vi "ODE_Template.vi"(0 "Reac Info":string[][](array[string])=[["Degradation_GFP", "", "false", "false", "Cell", "1", "GFP", "1.0", "true", "0", "", "", "0", "", "1", "kd", "0.0075"], ["Degradation_TetR", "", "false", "false", "Cell", "1", "TetR", "1.0", "true", "0", "", "", "0", "", "1", "kd", "0.0075"], ["Degradation_LacI", "", "false", "false", "Cell", "1", "LacI", "1.0", "true", "0", "", "", "0", "", "1", "kd", "0.0075"], ["R_abstracted_production_P1", "", "false", "false", "Cell", "0", "", "", "true", "1", "GFP", "10.0", "1", "LacI", "6", "RNAP, ng__P1, Ko__P1, ko__P1, nc__LacI_P1, Kr__LacI_P1", "30.0, 2.0, 0.033, 0.05, 2.0, 0.5"], ["R_abstracted_production_P2", "", "false", "false", "Cell", "0", "", "", "true", "1", "GFP", "10.0", "1", "TetR", "6", "RNAP, ng__P2, Ko__P2, ko__P2, nc__TetR_P2, Kr__TetR_P2", "30.0, 2.0, 0.033, 0.05, 2.0, 0.5"]], 1 "Ex_Mod_IDs":string[](array[string])=["LacI", "TetR"], 2 "Idx of Mod in Sp IDs":i32[](array[numeric])=[1, 4], 5 "Math Expressions":string[](array[string])=["kd*GFP", "kd*TetR", "kd*LacI", "ko__P1*ng__P1*Ko__P1*RNAP/(1+Ko__P1*RNAP+(Kr__LacI_P1*LacI)^nc__LacI_P1)", "ko__P2*ng__P2*Ko__P2*RNAP/(1+Ko__P2*RNAP+(Kr__TetR_P2*TetR)^nc__TetR_P2)"], 7 "Species Info":string[][](array[string])=[["GFP", "", "Cell", "0.0", "NaN", "", "true", "false", "false", "null"], ["LacI", "", "Cell", "0.0", "NaN", "", "true", "true", "false", "null"], ["P1", "", "Cell", "2.0", "NaN", "", "true", "false", "false", "null"], ["P2", "", "Cell", "2.0", "NaN", "", "true", "false", "false", "null"], ["TetR", "", "Cell", "0.0", "NaN", "", "true", "true", "false", "null"]], 9 "Parameter info":string[][](array[string])=[["ko_r", "Reverse RNAP binding rate", "1.0", "", "true"], ["nr", "Initial RNAP count", "30.0", "", "true"], ["np", "Stoichiometry of production", "10.0", "", "true"], ["kr_r", "Reverse repression binding rate", "1.0", "", "true"], ["ka_f", "Forward activation binding rate", "0.0033", "", "true"], ["kecdiff", "Extracellular diffusion rate", "1.0", "", "true"], ["ko", "Open complex production rate", "0.05", "", "true"], ["kmdiff_f", "Forward membrane diffusion rate", "1.0", "", "true"], ["kecd", "Extracellular degradation rate", "0.005", "", "true"], ["kc_r", "Reverse complex formation rate", "1.0", "", "true"], ["kr_f", "Forward repression binding rate", "0.5", "", "true"], ["ka_r", "Reverse activation binding rate", "1.0", "", "true"], ["nc", "Stoichiometry of binding", "2.0", "", "true"], ["kao_r", "Reverse activated RNAP binding rate", "1.0", "", "true"], ["kd", "Degradation rate", "0.0075", "", "true"], ["kb", "Basal production rate", "1.0E-4", "", "true"], ["ng", "Initial promoter count", "2.0", "", "true"], ["ka", "Activated production rate", "0.25", "", "true"], ["kao_f", "Forward activated RNAP binding rate", "1.0", "", "true"], ["kmdiff_r", "Reverse membrane diffusion rate", "0.01", "", "true"], ["ko_f", "Forward RNAP binding rate", "0.033", "", "true"], ["kc_f", "Forward complex formation rate", "0.05", "", "true"], ["High", "", "120.0", "", "true"], ["HighTime", "", "1000.0", "", "true"], ["HighTime2", "", "2000.0", "", "true"]], 11 "Local Parameter Info":string[][](array[string])=[["kd", "0.0075"], ["kd", "0.0075"], ["kd", "0.0075"], ["RNAP", "30.0"], ["ng__P1", "2.0"], ["Ko__P1", "0.033"], ["ko__P1", "0.05"], ["nc__LacI_P1", "2.0"], ["Kr__LacI_P1", "0.5"], ["RNAP", "30.0"], ["ng__P2", "2.0"], ["Ko__P2", "0.033"], ["ko__P2", "0.05"], ["nc__TetR_P2", "2.0"], ["Kr__TetR_P2", "0.5"]]) -> ()   [LabVIEW 2014]
uses:
  Modifier Control.ctl
  ODE Simulation Parameters.ctl
  <vilib>/Simulation/Implementation/Shared/SIM Continuous Solvers.ctl
  Event Info.ctl
  <vilib>/Utility/error.llb/DialogType.ctl
  Stop ODE.vi
  Sim status.vi
  Trigger Status Bar.vi
  <vilib>/Utility/file.llb/Write To Spreadsheet File (string).vi
  <vilib>/regexp/Match Regular Expression.xnode
panel:
  out "ScrSht Path":path
  out "loop":i32
  out "Rest_Sp_IDs":string[](array[string])
  out "Sp_Init_Amnt":string[](array[string])
  out "Fn Arg Cnt":string[](array[string])
  out "Functions":string[][](array[string])
  out "FuncCnt":i32
  out "Status update":string
  out "Trig Status":bool
  out "Comp IDs":string[](array[string])
  out "hasOnlySubstanceUnits":string[](array[string])
  out "Math-w/-ch-VarID":string[](array[string])
  out "LP_IDs":string[](array[string])
  out "Pr_Id_Arr":string[](array[string])
  out "Sp IDs":string[](array[string])
  out "Cap Cnt":i32
  out "Plot Legends":string[](array[string])
  out "ModTimeSym":string
  out "CompSize":string[](array[string])
  out "CompID":string[](array[string])
  out "Comp Def":string[][](array[string])
  out "Rules":string[][](array[string])
  out "RulesCnt":i32
  in  "Run":bool
  in  "Reset":bool
  in  "Stop Main":bool
  out "Sp_Name":string[](array[string])
  out "Nxt Sp State (N)":dbl[](array[numeric])
  out "T":dbl[](array[numeric])
  out "AppPath":string
  out "path":path
  in  "Shut Down":bool
  out "Sim Data":cluster{"times":dbl[], "outputs":dbl[][]}
  out "Rest_Sp_Init_Amnt":string[](array[string])
  in  "Simulation Parameters":T1={"Initial Time"=0.0, "Final Time"=20.0, "Time Step"=0.1, "Absolute Tolerance"=0.001, "Relative Tolerance"=1e-06, "Type of Continuous Solver"=enum."Runge-Kutta 45 (variable)", "Discrete Time Step"=2.0, "Minimum Time Step"=1e-06, "Maximum Time Step"=1.0, "Initial Time Step"=0.1} {"Initial Time Step" min=0.0; "Maximum Time Step" min=0.0; "Minimum Time Step" min=0.0; "Discrete Time Step" min=0.0; "Relative Tolerance" min=0.0; "Absolute Tolerance" min=0.0; "Time Step" min=0.0}
  in  "SP_for_ODE_Init_Amnt":string[](array[string])
  out "Out_X_for_ODE":string[](array[string])
  out "Out_Tot_Param":string[](array[string])
  out "Out_ODE":string[](array[string])
  in  "Model Name":string="nand_RB"
  out "Sp Ids":string[](array[string])
  out "XY Graph":cluster{"T":dbl[], dbl[]}[](graph)
  out "Nxt Sp State (S)":string[](array[string])
  out "Init Sp State (S)":string[](array[string])
  out "All Param Names":string[](array[string])
  out "Equations":string[](array[string])
  out "Init Sp State (N)":dbl[](array[numeric])
  out "All Param Vals":string[](array[string])
  out "All Param IDs":string[](array[string])
  out "New Total Pr IDs":string[](array[string])
  in  "Event Info":T3
  out "All Variables":string[](array[string])
  out "Math Assign":string[](array[string])
  out "Triggering Math":string[](array[string])
  in  "External Modifiers":T4[](array[typedef]) {"Dial" scale=0.0..100.0 scale format="%#_3g"}
  in  "Del events after \nexecution":bool
  in  "Capture Graph":bool caption="Save Data 2"
  in  "Save Data":bool
  in  "Sim Param":bool
  out "All Param Values":string[](array[string])
  out "Status":string
  in  "Events Info":string[][](table)=[["event0", "true", "true", "true", "t >= HighTime", "TetR = High"], ["event1", "true", "true", "true", "t >= HighTime2", "LacI = High"]]
  out "DataLog":path
  out "decimal integer string":string
  out "Horizontal Progress Bar":u8(slide) scale=0.0..100.0
  # "Virtual Laboratory Instrument for ODE Simulations"
  # "Powered By"
  # "Model Parameters"
  # "Global Parameters"
  # "Local Parameters"
  # "ID"
  # "Name"
  # "Value"
  # "ID"
  # "Value"
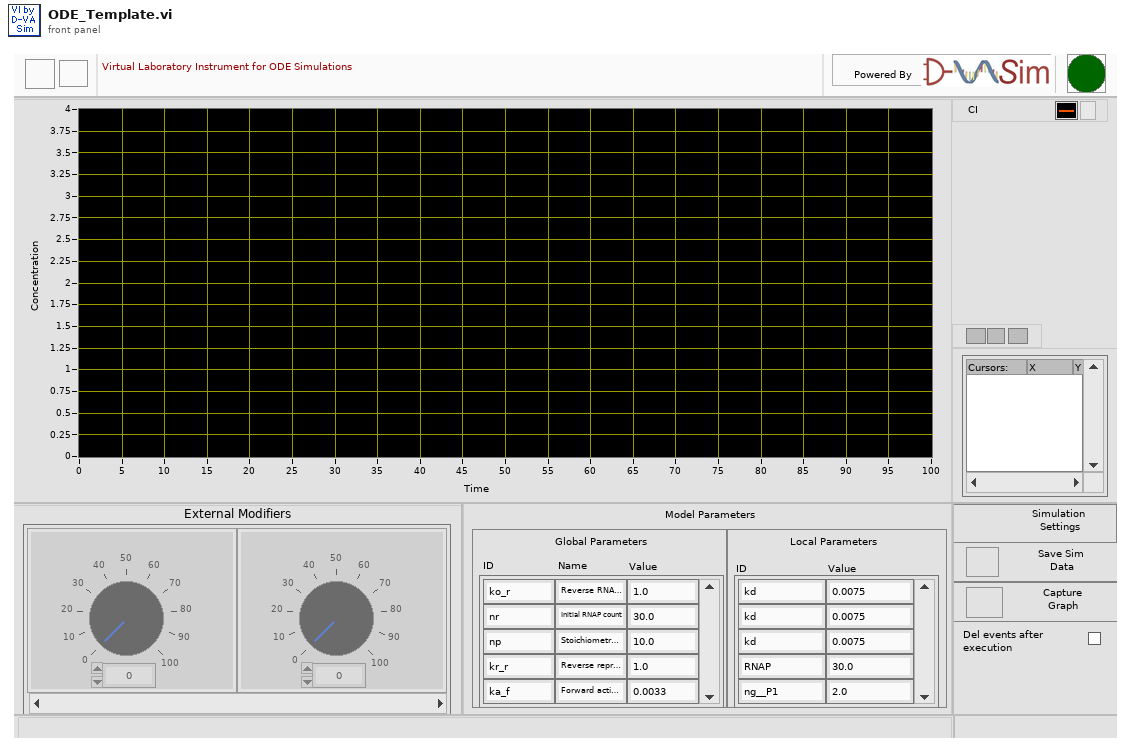
[diagram p1: front panel]
types:
  T1 = typedef "ODE Simulation Parameters.ctl" = cluster{"Initial Time":dbl, "Final Time":dbl, "Time Step":dbl, "Absolute Tolerance":dbl, "Relative Tolerance":dbl, "Type of Continuous Solver":T2, "Discrete Time Step":dbl, "Minimum Time Step":dbl, "Maximum Time Step":dbl, "Initial Time Step":dbl}
  T2 = typedef "SIM Continuous Solvers.ctl" = enum16{"Runge-Kutta 1 (Euler)", "Runge-Kutta 2", "Runge-Kutta 3", "Runge-Kutta 4", "Runge-Kutta 23 (variable)", "Runge-Kutta 45 (variable)", "BDF (variable)", "Adams-Moulton (variable)", "Rosenbrock (variable)", "Discrete States Only"}
  T3 = typedef "Event Info.ctl" = cluster{"Math Var":string[], "Math Op":string[], "Math Val":string[], "Assign Var":string[][], "Assign Op":string[][], "Assign Val":string[][], "Var Idx":i32[], "Assign Var Idx":i32[][], "Delay":string[], "Priority":string[]}
  T4 = typedef "Modifier Control.ctl" = cluster{"Dial":dbl, "String 2":string}
  T5 = enum8{"Enabled", "Disabled", "Disabled and Grayed Out"}
  T6 = typedef "DialogType.ctl" = u16
  T7 = typedef "Model Information.ctl" = cluster{"ID":string, "Name":string, "Substance Units":string, "Time Units":string, "Volume Units":string, "Area Units":string, "Length Units":string, "Extent Units":string, "Conversion Factor":string, "Model Components":string}
  T8 = cluster{"Model Info":T7, "SpCnt":i32, "Species Info":string[][], "Pr_Cnt":i32, "Parameter info":string[][], "ReacCnt":i32, "Reaction Info":string[][], "Math Expressions":string[][], "EventsCnt":i32, "Event Info":string[][], "UnitsDefCnt":i32, "Units Def":string[][], "CompCnt":i32, "Comp Def":string[][], "Mod_ID":string[], "Mod_Idx":i32[], "RulesCnt":i32, "Rules":string[][], "FuncCnt":i32, "Functions":string[][], "InitAssign Cnt":i32, "Init Assigns":string[][], "ConstraintsCnt":i32, "Constraints":string[][], "Fn Arg Cnt":string[]}
  T9 = cluster{"Reac Info":string[], "Reac Info":string[], "Reac Info":string[], "Math Expressions":string[], "Reac Info":string[], "Species Info":string[], "Sp IDs":string[], "Math-w/-ch-VarID":string[], "hasOnlySubstanceUnits":string[], "Comp IDs":string[]}
  T10 = cluster{"SP-for-ODE":string[], "Reac Info":string[], "Sp IDs":string[], "Species Info":string[], string[], "Reac Info":string[], "Reac Info":string[]}
  T11 = cluster{"Ex_Mod_IDs":string[], "Ex_Mod_IDs+Names":string[], "Ex_Mod_Init_Amnt":string[], "Rest_Sp_IDs ":string[], "Rest_Sp_IDs+Names":string[], "Rest_Sp_Init_Amnt":string[], "SP_for_ODE_Init_Amnt":string[], "Sp_for_ODE+Names":string[]}
  T12 = enum32{"invalid app kind", "Development System", "Run Time System", "Student Edition", "Embedded LabVIEW", "Evaluation", "Custom"}
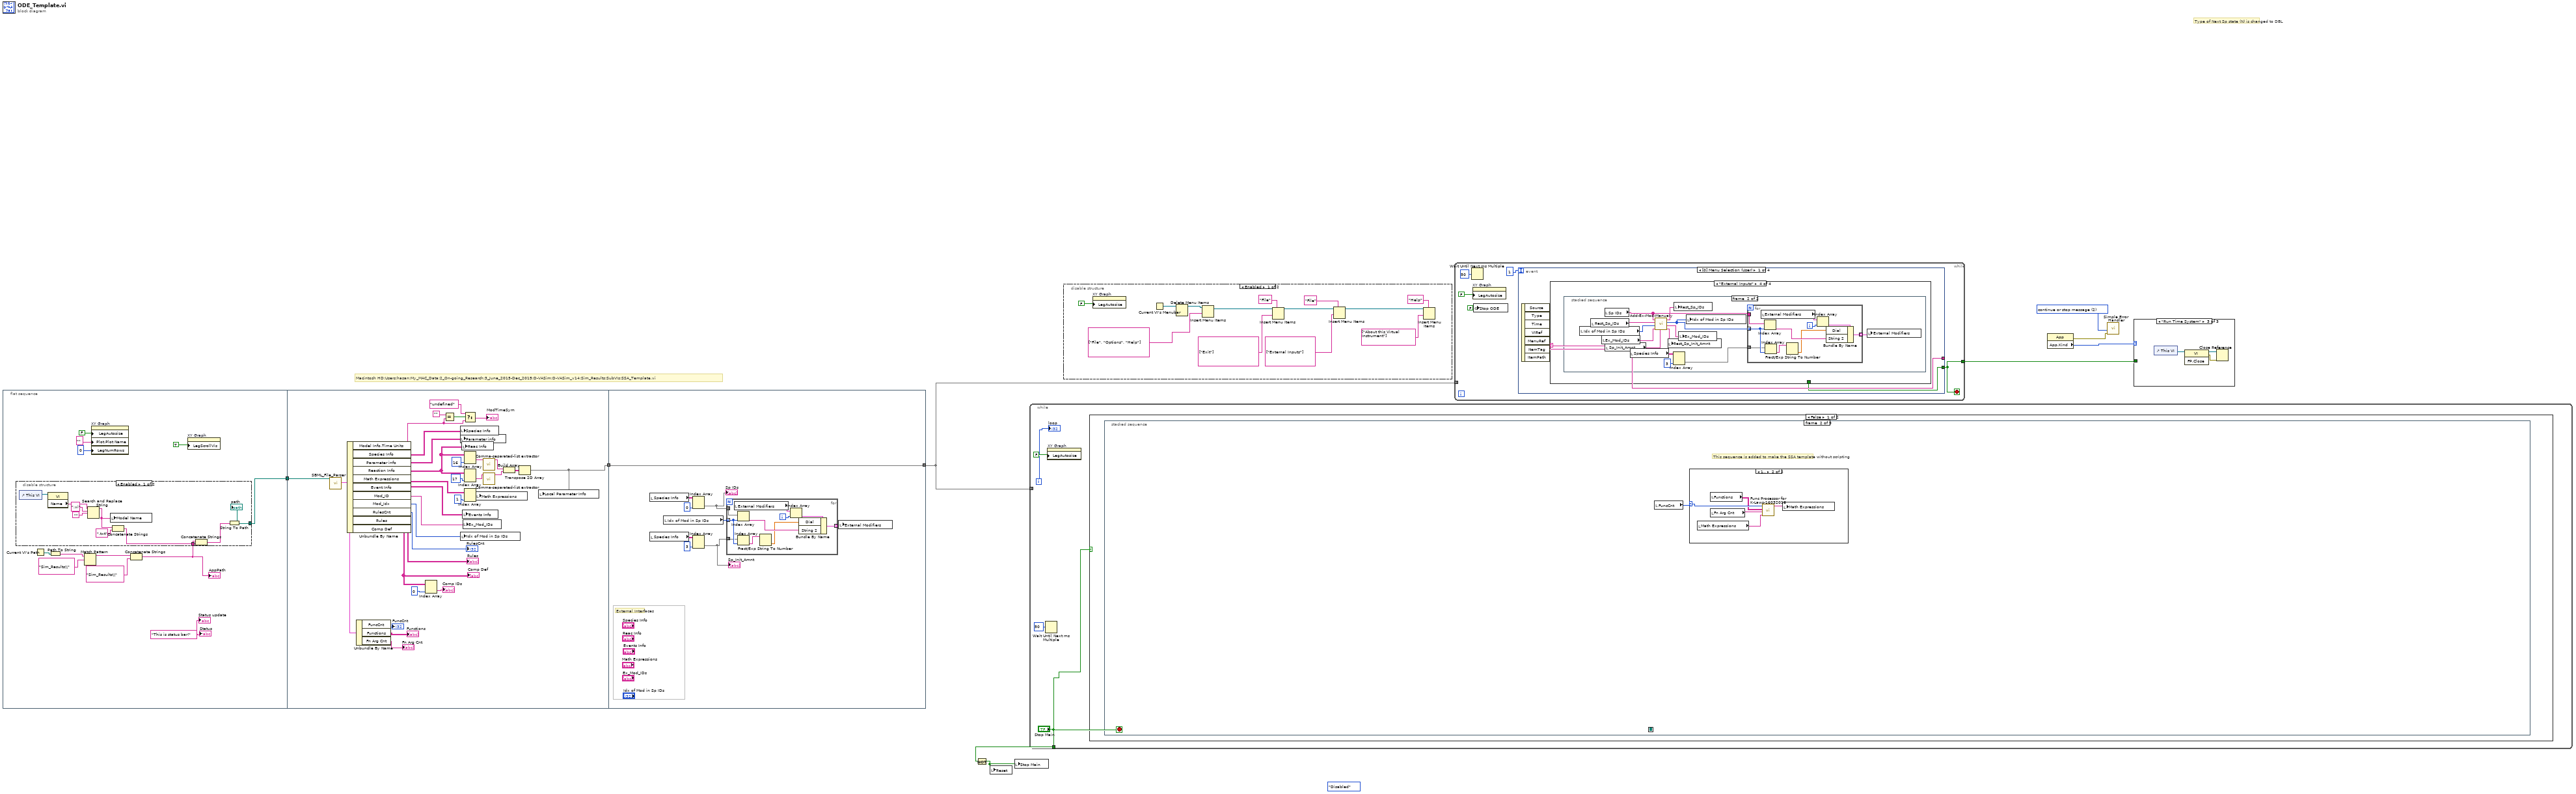
[diagram p0: block diagram]
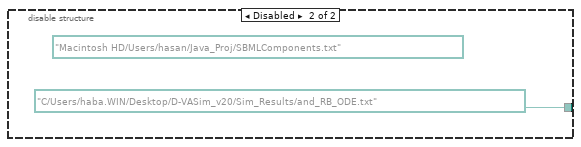
[diagram p2: hidden frame]
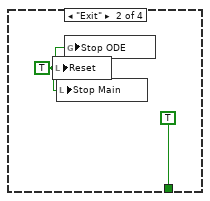
[diagram p7: hidden frame]
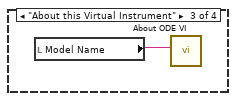
[diagram p8: hidden frame]
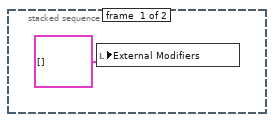
[diagram p9: hidden frame]
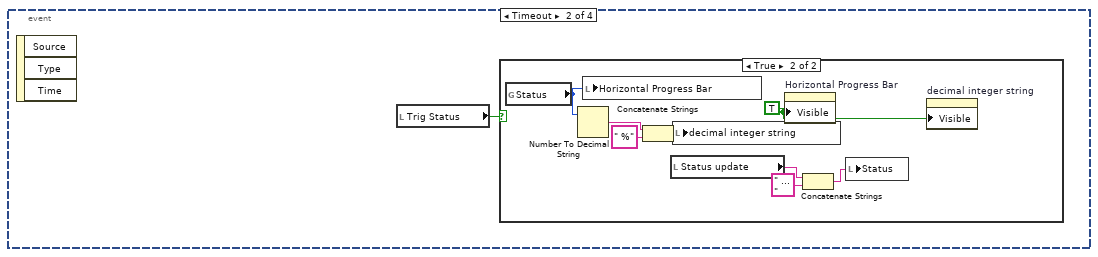
[diagram p10: hidden frame]
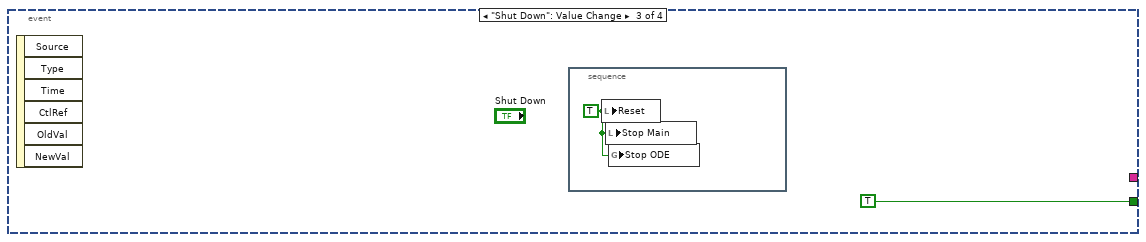
[diagram p12: hidden frame]
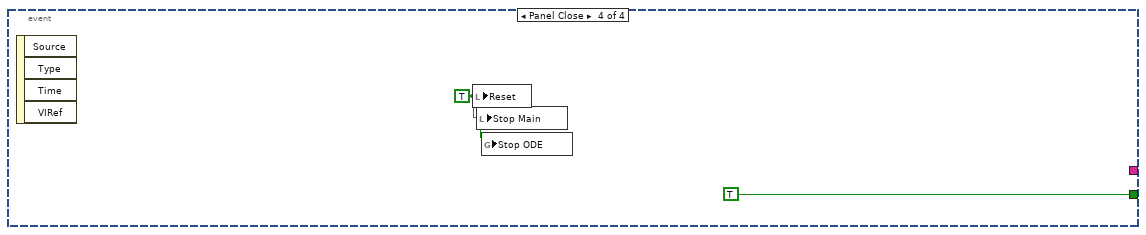
[diagram p13: hidden frame]
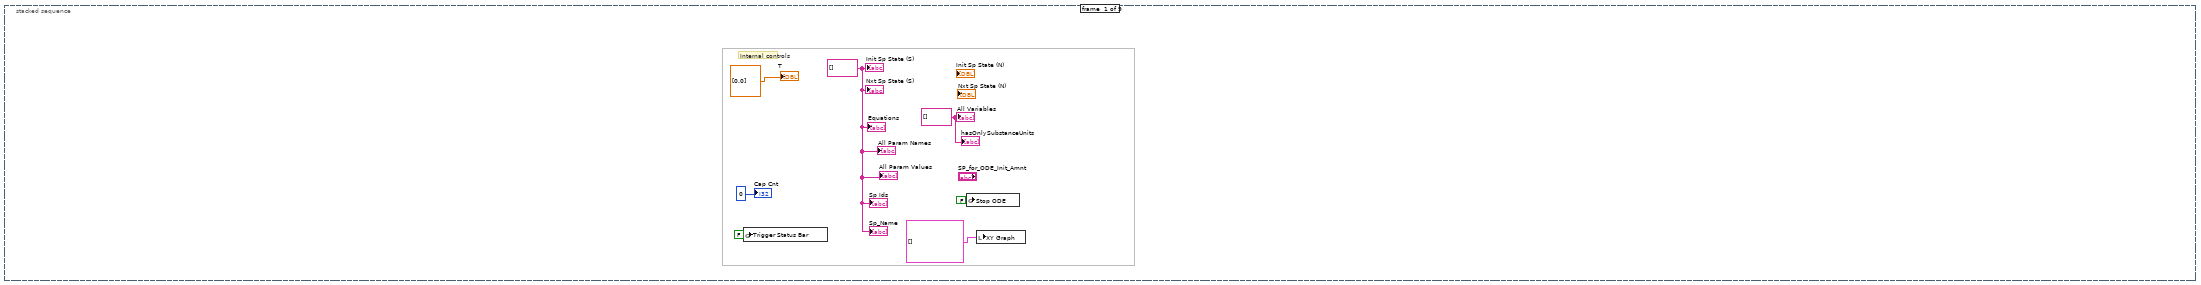
[diagram p14: hidden frame]
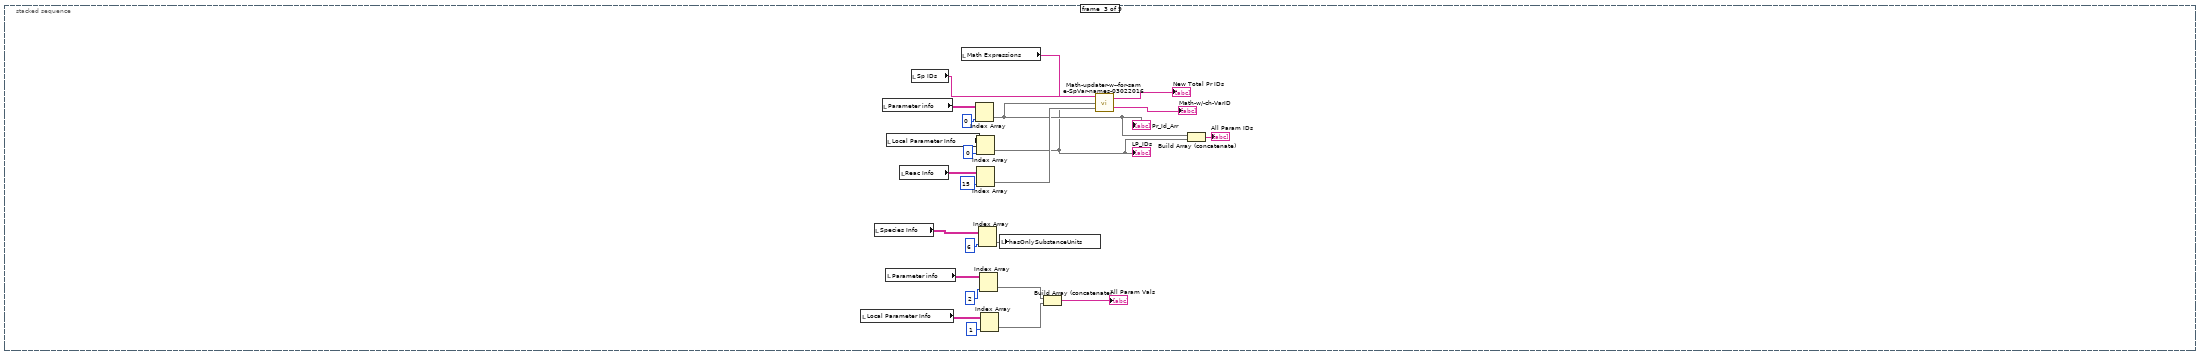
[diagram p16: hidden frame]
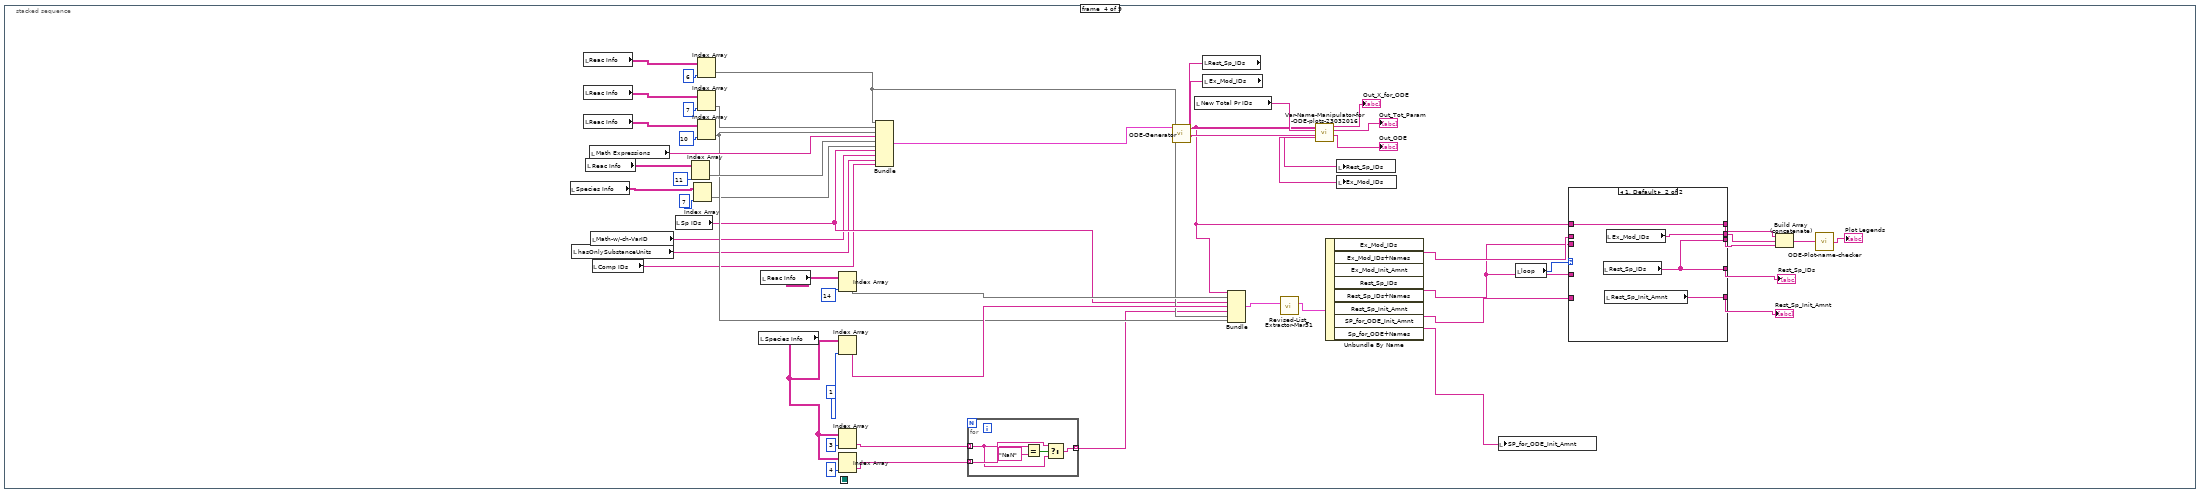
[diagram p17: hidden frame]
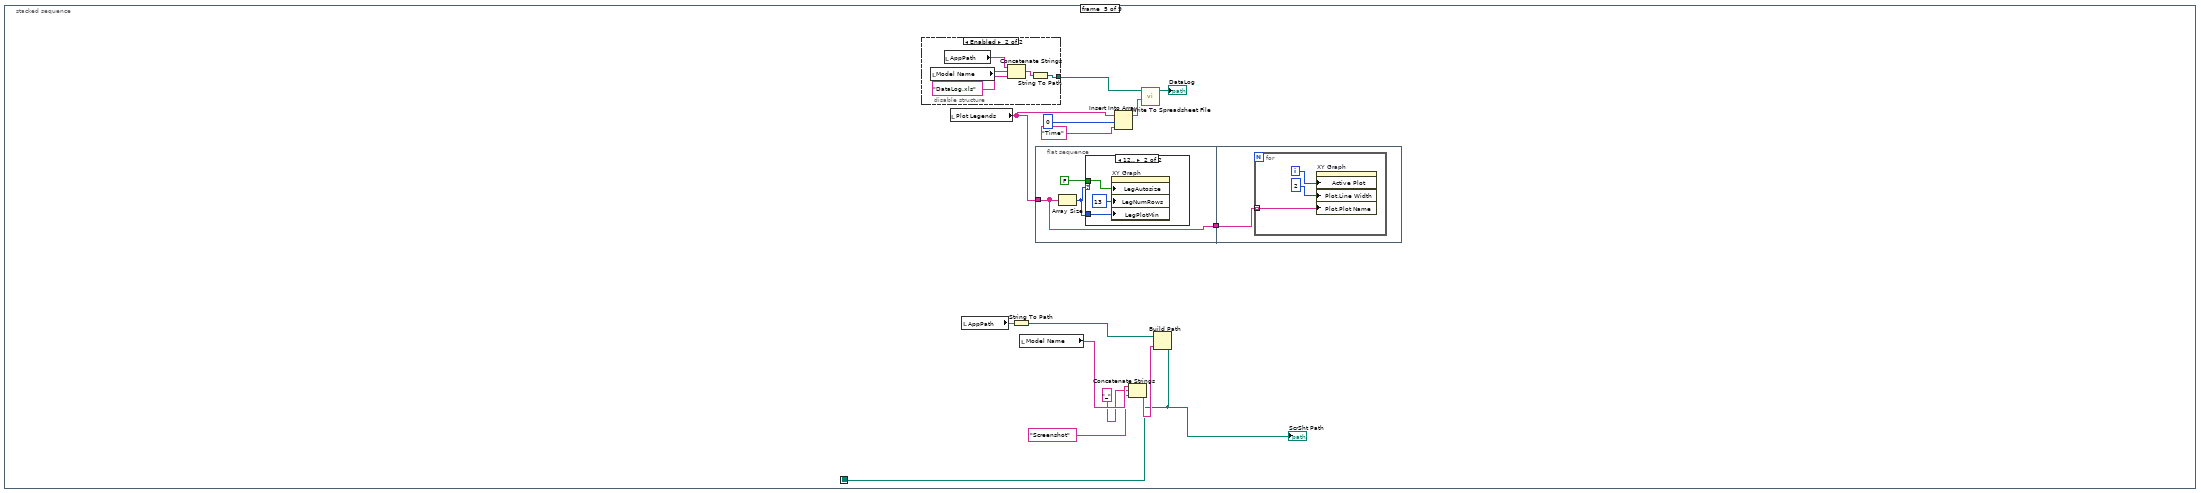
[diagram p19: hidden frame]
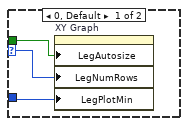
[diagram p20: hidden frame]
diagram:
  (unwired) T5."Disabled" ("Disabled")
  w8 = T6 2 items=["no dialog", "OK message", "continue or stop message", "OK message + warnings", "continue/stop + warnings"] ("type of dialog (OK msg:1)")
  # "Macintosh HD:Users:hasan:My_MAC_Data:2_On-going_Research:3_June_2015-Dec_2015:D-VASim:D-VASim_v14:Sim_Results:SubVIs:SSA_Template.vi"
  # "Type of Next Sp state (N) is changed to DBL"
  n1 = flat-sequence {
    tunnel: [w13] -> w2
    tunnel: w2 -> [w33]
    tunnel: [w38] -> w1
    tunnel: [w73] -> w3
    tunnel: w1 -> [w73]
    frame #0 {
      w21 = "This is status bar!" ("Status")
      n2 = Current VI's Path() -> (path=w15:path)
      n3 = Path To String(path=w15) -> (string=w16:string)
      n4 = Match Pattern(string=w16, regular expression="Sim_Results\\" ("string")) -> (before substring=w18:string)  [unwired: 1 in, 3 out]
      n5 = property on="XY Graph" class="XYGraph (strict)"("LegAutosize"=FALSE ("Legend:Scrollbar Visible"), "Plot.Plot Name"="", "LegNumRows"=u32 0 ("Legend:Number of Rows")) -> ()  [unwired: 2 in, 2 out]
      n6 = Concatenate Strings(w18, "Sim_Results\\" ("string")) -> (w20:string)
      "AppPath" <- w20
      n7 = disable-structure shown="Enabled" {
        disable-tunnel: [w31 path "C:/Users/haba.WIN/Desktop/D-VASim_v20/Sim_Results/and_RB_ODE.txt" ("SBML File")] -> w13
        disable-tunnel: w20 -> [w22 _]
        frame Enabled {
          n8 = control-ref of="This VI"() -> (w30:refnum<vi>)
          n9 = property class="VI"(reference=w30) -> ("Name"=w29:string)  [unwired: 1 in, 2 out]
          n10 = Search and Replace String(input string=w29, search string=".vi", replace string="") -> (result string=w26:string)  [unwired: 5 in, 3 out]
          n11 = local write "Model Name"(w26) -> ()
          n12 = Concatenate Strings(w26, ".txt" ("search string")) -> (w24:string)
          n13 = Concatenate Strings(w22, w24) -> (w23:string)
          n14 = String To Path(string=w23) -> (path=w31:path)
          "path" <- w31
        }
        frame Disabled {
          (unwired) path "/Macintosh HD/Users/hasan/Java_Proj/SBMLComponents.txt" ("SBML File")
        }
      }
      n15 = property on="XY Graph" class="XYGraph (strict)"("LegScrollVis"=TRUE ("Legend:Scrollbar Visible")) -> ()  [unwired: 2 in, 2 out]
      "Status update" <- w21
      "Status" <- w21
    }
    frame #1 {
      n16 = call "SBML_File_Parser.vi"("SBML File"=w33) -> ("SBML Data"=w37:T8)  [unwired: 17 in, 1 out]
      n17 = Unbundle By Name(w37) -> ("Model Info.Time Units"=w43:string, "Species Info"=w58:string[][], "Parameter info"=w57:string[][], "Reaction Info"=w56:string[][], "Math Expressions"=w53:string[][], "Event Info"=w51:string[][], "Mod_ID"=w50:string[], "Mod_Idx"=w49:i32[], "RulesCnt"=→"RulesCnt":i32, "Rules"=→"Rules":string[][], "Comp Def"=w40:string[][])
      "Comp Def" <- w40
      n18 = Unbundle By Name(w37) -> ("FuncCnt"=→"FuncCnt":i32, "Functions"=→"Functions":string[][], "Fn Arg Cnt"=→"Fn Arg Cnt":string[])
      n19 = Index Array(array=w40, index (col)=0 ("disabled index (col)")) -> (element=→"Comp IDs":string[])  [unwired: 1 in]
      n20 = Equal?(x="", y=w43) -> (x = y?=w45:bool)
      n21 = local write "Species Info"(w58) -> ()
      n22 = local write "Parameter info"(w57) -> ()
      n23 = local write "Idx of Mod in Sp IDs"(w49) -> ()
      n24 = local write "Reac Info"(w56) -> ()
      n25 = local write "Events Info"(w51) -> ()
      n26 = local write "Ex_Mod_IDs"(w50) -> ()
      n27 = Select(t="undefined", s=w45, f=w43) -> (s? t:f=→"ModTimeSym":string)
      n28 = Index Array(array=w56, index (col)=17 ("disabled index (col)")) -> (element=w54:string[])  [unwired: 1 in]
      n29 = Index Array(array=w53, index (col)=1 ("disabled index (col)")) -> (element=w52:string[])  [unwired: 1 in]
      n30 = Index Array(array=w56, index (col)=16 ("disabled index (col)")) -> (element=w55:string[])  [unwired: 1 in]
      n31 = local write "Math Expressions"(w52) -> ()
      n32 = call "Comma-separated-list extractor.vi"("In_list"=w55) -> ("List_Out"=w60:string[])  [unwired: 6 in, 1 out]
      n33 = call "Comma-separated-list extractor.vi"("In_list"=w54) -> ("List_Out"=w59:string[])  [unwired: 6 in, 1 out]
      n34 = Build Array(w60, w59) -> (w61:string[][])
      n35 = Transpose 2D Array(2D array=w61) -> (transposed array=w38:string[][])
      n36 = local write "Local Parameter Info"(w38) -> ()
    }
    frame #2 {
      # "External Interfaces"
      n37 = local read "Species Info"() -> (w66:string[][])
      n38 = local read "Species Info"() -> (w71:string[][])
      n39 = local read "Idx of Mod in Sp IDs"() -> (w69:i32[])
      n40 = Index Array(array=w66, index (col)=0 ("disabled index (col)")) -> (element=w72:string[])  [unwired: 1 in]
      "Sp IDs" <- w72
      n41 = Index Array(array=w71, index (col)=3 ("disabled index (col)")) -> (element=w65:string[])  [unwired: 1 in]
      "Sp_Init_Amnt" <- w65
      n42 = for {
        tunnel: w69 -> [w77] mode=indexing
        tunnel: w72 -> [w83]
        tunnel: [w79] -> w68 mode=indexing
        tunnel: w65 -> [w76]
        i -> [w81]
        n43 = local read "External Modifiers"() -> (w82:T4[])
        n44 = Index Array(array=w83, index=w77) -> (element=w78:string)
        n45 = Index Array(array=w76, index=w77) -> (element=w75:string)
        n46 = Fract/Exp String To Number(string=w75) -> (number=w74:dbl)  [unwired: 3 in, 1 out]
        n47 = Index Array(array=w82, index=w81) -> (element=w80:T4)
        n48 = Bundle By Name(cluster=w80, "Dial"=w74, "String 2"=w78) -> (w79:T4)
      }
      n49 = local write "External Modifiers"(w68) -> ()
    }
  }
  n50 = while {
    tunnel: ["Stop Main"] -> w5
    tunnel: w3 -> [_]
    i -> [w84]
    stop <- "Stop Main" stop-if-true
    n51 = Wait Until Next ms Multiple(millisecond multiple=u32 50) -> ()  [unwired: 1 out]
    n52 = property on="XY Graph" class="XYGraph (strict)"("LegAutosize"=FALSE ("Legend:Scrollbar Visible")) -> ()  [unwired: 2 in, 2 out]
    n53 = case shown="False" "Stop Main" {
      frame False {
        n54 = stacked-sequence {
          seq-local: [_ _ _ _ w195 _ _ _ _] -> [_ _ _ _ _ _ _ _ w561]
          frame #0 {
            w90 = string[] [] ("All Variables")
            w92 = string[] [] ("Init Sp State (S)")
            # "Internal controls"
            n55 = global write "Trigger Status Bar.vi" "Trigger Status Bar"(FALSE ("Trigger Status Bar 2")) -> ()
            n56 = global write "Stop ODE.vi" "Stop ODE"(FALSE ("Stop ODE")) -> ()
            n57 = local write "XY Graph"(cluster{"T":dbl[], dbl[]}[] [] ("XY Graph")) -> ()
            "Equations" <- w92
            "T" <- dbl[] [0.0] ("T")
            "Nxt Sp State (S)" <- w92
            "Init Sp State (S)" <- w92
            "Sp Ids" <- w92
            "Sp_Name" <- w92
            "All Param Names" <- w92
            "All Param Values" <- w92
            "Cap Cnt" <- 0 ("Cap Cnt")
            "All Variables" <- w90
            "hasOnlySubstanceUnits" <- w90
          }
          frame #1 {
            # "This sequence is added to make the SSA template without scripting"
            n58 = local read "FuncCnt"() -> (w95:i32)
            n59 = case shown="1.." w95 {
              selector: w95 -> [_ w100]
              frame 0, Default {
              }
              frame 1.. {
                n60 = local read "Math Expressions"() -> (w99:string[])
                n61 = local read "Functions"() -> (w97:string[][])
                n62 = local read "Fn Arg Cnt"() -> (w96:string[])
                n63 = call "Func Processor for K-Laws-16032016.vi"("Math Expressions In"=w99, "Fn Arg Cnt"=w96, "Functions Definition"=w97, "Total Function Definitions"=w100) -> ("Math Expressions Out"=w98:string[])  [unwired: 7 in]
                n64 = local write "Math Expressions"(w98) -> ()
              }
            }
          }
          frame #2 {
            n65 = local read "Local Parameter Info"() -> (w109:string[][])
            n66 = local read "Species Info"() -> (w122:string[][])
            n67 = local read "Parameter info"() -> (w118:string[][])
            n68 = local read "Parameter info"() -> (w108:string[][])
            n69 = local read "Local Parameter Info"() -> (w117:string[][])
            n70 = local read "Reac Info"() -> (w123:string[][])
            n71 = local read "Sp IDs"() -> (w101:string[])
            n72 = local read "Math Expressions"() -> (w116:string[])
            n73 = Index Array(array=w118, index (col)=0 ("disabled index (col)")) -> (element=w112:string[])  [unwired: 1 in]
            "Pr_Id_Arr" <- w112
            n74 = Index Array(array=w117, index (col)=0 ("disabled index (col)")) -> (element=w111:string[])  [unwired: 1 in]
            "LP_IDs" <- w111
            n75 = Index Array(array=w123, index (col)=15 ("disabled index (col)")) -> (element=w115:string[])  [unwired: 1 in]
            n76 = Index Array(array=w122, index (col)=6 ("disabled index (col)")) -> (element=w102:string[])  [unwired: 1 in]
            n77 = Index Array(array=w108, index (col)=2 ("disabled index (col)")) -> (element=w105:string[])  [unwired: 1 in]
            n78 = Index Array(array=w109, index (col)=1 ("disabled index (col)")) -> (element=w104:string[])  [unwired: 1 in]
            n79 = local write "hasOnlySubstanceUnits"(w102) -> ()
            n80 = Build Array (concatenate)(w105, w104) -> (→"All Param Vals":string[])
            n81 = call "Math-updater-w--for-same-SpVar-names-03022016.vi"("Sp_Id_Arr"=w101, "Math Expressions"=w116, "Pr_Id_Arr"=w112, "LP-Cnt_4_Reac"=w115, "LP_IDs"=w111) -> ("New Total Pr IDs"=→"New Total Pr IDs":string[], "Math-w/-ch-VarID"=→"Math-w/-ch-VarID":string[])
            n82 = Build Array (concatenate)(w112, w111) -> (→"All Param IDs":string[])
          }
          frame #3 {
            n83 = local read "Species Info"() -> (w154:string[][])
            n84 = local read "hasOnlySubstanceUnits"() -> (w149:string[])
            n85 = local read "Reac Info"() -> (w179:string[][])
            n86 = local read "Reac Info"() -> (w178:string[][])
            n87 = local read "Reac Info"() -> (w174:string[][])
            n88 = local read "Reac Info"() -> (w167:string[][])
            n89 = local read "Math Expressions"() -> (w172:string[])
            n90 = local read "Math-w/-ch-VarID"() -> (w150:string[])
            n91 = local read "Comp IDs"() -> (w148:string[])
            n92 = local read "Sp IDs"() -> (w153:string[])
            n93 = Index Array(array=w167, index (col)=11 ("disabled index (col)")) -> (element=w173:string[])  [unwired: 1 in]
            n94 = Index Array(array=w154, index (col)=7 ("disabled index (col)")) -> (element=w155:string[])  [unwired: 1 in]
            n95 = Index Array(array=w179, index (col)=6 ("disabled index (col)")) -> (element=w163:string[])  [unwired: 1 in]
            n96 = Index Array(array=w178, index (col)=7 ("disabled index (col)")) -> (element=w176:string[])  [unwired: 1 in]
            n97 = Index Array(array=w174, index (col)=10 ("disabled index (col)")) -> (element=w162:string[])  [unwired: 1 in]
            n98 = local read "Species Info"() -> (w143:string[][])
            n99 = local read "Reac Info"() -> (w158:string[][])
            n100 = Index Array(array=w158, index (col)=14 ("disabled index (col)")) -> (element=w166:string[])  [unwired: 1 in]
            n101 = Index Array(array=w143, index (col)=1 ("disabled index (col)")) -> (element=w164:string[])  [unwired: 1 in]
            n102 = Index Array(array=w143, index (col)=3 ("disabled index (col)")) -> (element=w146:string[])  [unwired: 1 in]
            n103 = Index Array(array=w143, index (col)=4 ("disabled index (col)")) -> (element=w142:string[])  [unwired: 1 in]
            n104 = Bundle("Reac Info"=w163, "Reac Info"=w176, "Reac Info"=w162, "Math Expressions"=w172, "Reac Info"=w173, "Species Info"=w155, "Sp IDs"=w153, "Math-w/-ch-VarID"=w150, "hasOnlySubstanceUnits"=w149, "Comp IDs"=w148) -> (w147:T9)  [unwired: 1 in]
            n105 = for {
              tunnel: w146 -> [w191] mode=indexing
              tunnel: w142 -> [w192] mode=indexing
              tunnel: [w190] -> w141 mode=indexing
              n106 = Equal?(x=w191, y="NaN") -> (x = y?=w193:bool)
              n107 = Select(t=w192, s=w193, f=w191) -> (s? t:f=w190:string)
            }
            n108 = call "ODE-Generator.vi"("Cluster"=w147) -> ("Final ODE 2"=w151:string[], "SP-for-ODE"=w134:string[])  [unwired: 5 in, 2 out]
            n109 = local read "New Total Pr IDs"() -> (w152:string[])
            n110 = local read "Rest_Sp_IDs"() -> (w137:string[])
            n111 = local read "Ex_Mod_IDs"() -> (w138:string[])
            n112 = Bundle("SP-for-ODE"=w134, "Reac Info"=w166, "Sp IDs"=w153, "Species Info"=w164, w141, "Reac Info"=w163, "Reac Info"=w162) -> (w161:T10)  [unwired: 1 in]
            n113 = call "Revised-List_Extractor-Mar31.vi"("Input Cluster"=w161) -> ("Output Cluster"=w160:T11)  [unwired: 13 in, 1 out]
            n114 = call "Var-Name-Manipulator-for-ODE-plots-23032016.vi"("In_Rest_Sp_IDs"=w137, "In_Ex_Mod_IDs"=w138, "In_ODE"=w151, "In_Tot_Param"=w152, "In_X_for_ODE"=w134) -> ("Out_ODE"=→"Out_ODE":string[], "Out_Tot_Param"=→"Out_Tot_Param":string[], "Out_X_for_ODE"=→"Out_X_for_ODE":string[], "Out_Rest_Sp_IDs"=w136:string[], "Out_Ex_Mod_IDs"=w135:string[])  [unwired: 1 in, 1 out]
            n115 = Unbundle By Name(w160) -> ("Ex_Mod_IDs"=w133:string[], "Rest_Sp_IDs"=w125:string[], "Rest_Sp_Init_Amnt"=w127:string[], "SP_for_ODE_Init_Amnt"=w159:string[])  [unwired: 4 out]
            n116 = local write "Rest_Sp_IDs"(w136) -> ()
            n117 = local write "Ex_Mod_IDs"(w135) -> ()
            n118 = local write "SP_for_ODE_Init_Amnt"(w159) -> ()
            n119 = local read "loop"() -> (w132:i32)
            n120 = case shown="1, Default" w132 {
              tunnel: w134 -> [w185 w189]
              tunnel: w133 -> [w184 _]
              tunnel: w125 -> [w183 _]
              tunnel: [w185 w189] -> w131
              tunnel: [w184 w188] -> w130
              tunnel: [w183 w186] -> w129
              tunnel: [w182 w187] -> w128
              tunnel: w127 -> [w182 _]
              tunnel: [w181 w186] -> w126
              tunnel: w125 -> [w181 _]
              frame 0 {
              }
              frame 1, Default {
                n121 = local read "Rest_Sp_IDs"() -> (w186:string[])
                n122 = local read "Rest_Sp_Init_Amnt"() -> (w187:string[])
                n123 = local read "Ex_Mod_IDs"() -> (w188:string[])
              }
            }
            "Rest_Sp_Init_Amnt" <- w128
            "Rest_Sp_IDs" <- w126
            n124 = Build Array (concatenate)(w131, w130, w129) -> (w140:string[])
            n125 = call "ODE-Plot-name-checker.vi"("In Plot Name"=w140) -> ("Out Plot Name"=→"Plot Legends":string[])
          }
          frame #4 {
            n126 = disable-structure shown="Enabled" {
              disable-tunnel: [w222 w232] -> w200
              frame Disabled {
                n127 = call <vilib>:"Application Directory.vi"() -> ("Application Directory"=w224:path)
                n128 = Path To String(path=w224) -> (string=w225:string)
                n129 = Concatenate Strings(w225, ":Sim_Results:", "Model Name") -> (w226:string)
                n130 = String To Path(string=w226) -> (path=w222:path)
              }
              frame Enabled {
                n131 = local read "Model Name"() -> (w229:string)
                n132 = local read "AppPath"() -> (w231:string)
                n133 = Concatenate Strings(w231, w229, "DataLog.xls") -> (w228:string)
                n134 = String To Path(string=w228) -> (path=w232:path)
              }
            }
            n135 = local read "Plot Legends"() -> (w197:string[])
            n136 = local read "AppPath"() -> (w199:string)
            n137 = String To Path(string=w199) -> (path=w198:path)
            n138 = local read "Model Name"() -> (w204:string)
            n139 = flat-sequence {
              tunnel: w197 -> [w209]
              tunnel: [w209] -> w196
              tunnel: w196 -> [w218]
              frame #0 {
                n140 = Array Size(array=w209) -> (size(s)=w210:i32)
                n141 = case shown="12.." w210 {
                  selector: w210 -> [w213 _]
                  tunnel: FALSE ("Legend:Autosize") -> [w214 w217]
                  tunnel: w210 -> [w212 w215]
                  frame 0, Default {
                    n142 = property on="XY Graph" class="XYGraph (strict)"("LegAutosize"=w214, "LegNumRows"=w213, "LegPlotMin"=w212) -> ()  [unwired: 2 in, 2 out]
                  }
                  frame 12.. {
                    n143 = property on="XY Graph" class="XYGraph (strict)"("LegAutosize"=w217, "LegNumRows"=u32 13 ("Legend:Number of Rows"), "LegPlotMin"=w215) -> ()  [unwired: 2 in, 2 out]
                  }
                }
              }
              frame #1 {
                n144 = for {
                  tunnel: w218 -> [w219] mode=indexing
                  i -> [w221]
                  n145 = property on="XY Graph" class="XYGraph (strict)"("Active Plot"=w221, "Plot.Line Width"=u8 2, "Plot.Plot Name"=w219) -> ()  [unwired: 2 in, 2 out]
                }
              }
            }
            n146 = Insert Into Array(array=w197, index=0, new element="Time" ("string")) -> (w206:string[])
            n147 = Concatenate Strings(w204, "_" ("string"), "Screenshot" ("name or relative path")) -> (w201:string)
            n148 = call-poly <vilib>:"Write To Spreadsheet File.vi"("1D data"=w206, "file path (dialog if empty)"=w200) -> ("new file path (Not A Path if cancelled)"=→"DataLog":path)  [unwired: 6 in]
            n149 = Build Path(base path=w198, name or relative path=w201) -> (appended path=w195:path)
            "ScrSht Path" <- w195
          }
          frame #5 {
            n150 = disable-structure shown="Enabled" {
              frame Disabled {
                n151 = local read "Species Info"() -> (w241:string[][])
                n152 = Index Array(array=w241, index (col)=3 ("disabled index (col)")) -> (element=w240:string[])  [unwired: 1 in]
                n153 = local write "Init Sp State (S)"(w240) -> ()
                n154 = Fract/Exp String To Number(string=w240) -> (number=w239:dbl[])  [unwired: 3 in, 1 out]
                n155 = local write "Init Sp State (N)"(w239) -> ()
                n156 = local write "Nxt Sp State (N)"(w239) -> ()
                n157 = Number To Fractional String(number=w239) -> (F-format string=w238:string[])  [unwired: 3 in]
                n158 = local write "Nxt Sp State (S)"(w238) -> ()
              }
              frame Enabled {
              }
            }
            n159 = local read "Comp Def"() -> (w235:string[][])
            n160 = Index Array(array=w235, index (col)=0 ("disabled index (col)")) -> (element=→"CompID":string[])  [unwired: 1 in]
            n161 = Index Array(array=w235, index (col)=3 ("disabled index (col)")) -> (element=→"CompSize":string[])  [unwired: 1 in]
          }
          frame #6 {
            # "Gatheriing all the variables in a single array"
            n162 = local read "Plot Legends"() -> (w243:string[])
            n163 = local read "CompID"() -> (w245:string[])
            n164 = Build Array (concatenate)(string[] ["t"] ("array"), w243, w245) -> (w246:string[])
            n165 = local write "All Variables"(w246) -> ()
          }
          frame #7 {
            # "Processing SBML Events"
            n166 = local read "Events Info"() -> (w258:string[][])
            n167 = Index Array(array=w258, index (col)=4 ("disabled index (col)")) -> (element=w250:string[])  [unwired: 1 in]
            "Triggering Math" <- w250
            n168 = Index Array(array=w258, index (col)=5 ("disabled index (col)")) -> (element=w248:string[])  [unwired: 1 in]
            "Math Assign" <- w248
            n169 = Index Array(array=w258, index (col)=6 ("disabled index (col)")) -> (element=w257:string[])  [unwired: 1 in]
            n170 = Index Array(array=w258, index (col)=7 ("disabled index (col)")) -> (element=w256:string[])  [unwired: 1 in]
            n171 = local read "FuncCnt"() -> (w251:i32)
            n172 = case shown="1.." w251 {
              selector: w251 -> [_ w277]
              tunnel: w250 -> [w270 w274]
              tunnel: [w270 w273] -> w249
              tunnel: w248 -> [w269 w272]
              tunnel: [w269 w271] -> w247
              frame 0, Default {
              }
              frame 1.. {
                n173 = local read "Fn Arg Cnt"() -> (w275:string[])
                n174 = local read "Functions"() -> (w276:string[][])
                n175 = call "Func Processor for Events.vi"("Math Assign In"=w272, "Triggering Math In"=w274, "Fn Arg Cnt"=w275, "Functions Definition"=w276, "Total Function Definitions"=w277) -> ("Math Assign Out"=w271:string[], "Triggering Math Out"=w273:string[])  [unwired: 5 in]
              }
            }
            n176 = for {
              tunnel: w249 -> [w303] mode=indexing
              tunnel: [w293] -> w262 mode=indexing
              tunnel: [w285] -> w265 mode=indexing
              tunnel: [w295] -> w266 mode=indexing
              tunnel: [w292] -> w261 mode=indexing
              tunnel: [w284] -> w255 mode=indexing
              tunnel: [w283] -> w254 mode=indexing
              tunnel: [w282] -> w253 mode=indexing
              tunnel: [w281] -> w252 mode=indexing
              tunnel: w247 -> [w279] mode=indexing
              n177 = Build Array(w279) -> (w278:string[])
              n178 = call "Comma-separated-list extractor.vi"("In_list"=w278) -> ("List_Out"=w280:string[])  [unwired: 6 in, 1 out]
              n179 = xnode "Match Regular Expression"("input string"=w303, "regular expression"="[><][=]|>|<") -> ("before match"=w301:string, "whole match"=w295:string, "after match"=w296:string)  [unwired: 4 in, 2 out]
              n180 = call <vilib>:"Space Constant.vi"() -> ("String"=w298:string)
              n181 = call <vilib>:"Space Constant.vi"() -> ("String"=w300:string)
              n182 = Search and Replace String(input string=w296, search string=w298, replace string="") -> (result string=w287:string)  [unwired: 5 in, 3 out]
              n183 = Search and Replace String(input string=w301, search string=w300, replace string="") -> (result string=w293:string)  [unwired: 5 in, 3 out]
              n184 = local read "All Param IDs"() -> (w286:string[])
              n185 = Search 1D Array(1D array=w286, element=w287) -> (index of element=w289:i32)  [unwired: 1 in]
              n186 = for {
                tunnel: [w311] -> w284 mode=indexing
                tunnel: [w310] -> w283 mode=indexing
                tunnel: [w309] -> w282 mode=indexing
                tunnel: [w308] -> w281 mode=indexing
                tunnel: w280 -> [w304] mode=indexing
                n187 = xnode "Match Regular Expression"("input string"=w304, "regular expression"="=") -> ("before match"=w316:string, "whole match"=w309:string, "after match"=w322:string)  [unwired: 4 in, 2 out]
                n188 = call <vilib>:"Space Constant.vi"() -> ("String"=w320:string)
                n189 = call <vilib>:"Space Constant.vi"() -> ("String"=w315:string)
                n190 = Search and Replace String(input string=w322, search string=w320, replace string="") -> (result string=w305:string)  [unwired: 5 in, 3 out]
                n191 = Search and Replace String(input string=w316, search string=w315, replace string="") -> (result string=w310:string)  [unwired: 5 in, 3 out]
                n192 = local read "All Param IDs"() -> (w319:string[])
                n193 = Search 1D Array(1D array=w319, element=w305) -> (index of element=w306:i32)  [unwired: 1 in]
                n194 = case shown="1" w306 {
                  selector: w306 -> [_ w324]
                  tunnel: [w323 w325] -> w307
                  tunnel: w305 -> [w323 _]
                  frame 0, Default {
                  }
                  frame 1 {
                    n195 = local read "All Param Vals"() -> (w326:string[])
                    n196 = Index Array(array=w326, index=w324) -> (element=w325:string)
                  }
                }
                n197 = call <vilib>:"Space Constant.vi"() -> ("String"=w313:string)
                n198 = Search and Replace String(input string=w307, search string=w313, replace string="") -> (result string=w308:string)  [unwired: 5 in, 3 out]
                n199 = local read "All Variables"() -> (w318:string[])
                n200 = Search 1D Array(1D array=w318, element=w310) -> (index of element=w311:i32)  [unwired: 1 in]
              }
              n201 = case shown="0, Default" w289 {
                selector: w289 -> [w442 _]
                tunnel: [w441 w444] -> w288
                tunnel: w287 -> [_ w444]
                frame 0, Default {
                  n202 = local read "All Param Vals"() -> (w443:string[])
                  n203 = Index Array(array=w443, index=w442) -> (element=w441:string)
                }
                frame -1 {
                }
              }
              n204 = call <vilib>:"Space Constant.vi"() -> ("String"=w291:string)
              n205 = Search and Replace String(input string=w288, search string=w291, replace string="") -> (result string=w285:string)  [unwired: 5 in, 3 out]
              n206 = local read "All Variables"() -> (w294:string[])
              n207 = Search 1D Array(1D array=w294, element=w293) -> (index of element=w292:i32)  [unwired: 1 in]
            }
            n208 = Bundle By Name(cluster="Event Info", "Math Var"=w262, "Math Op"=w266, "Math Val"=w265, "Assign Var"=w254, "Assign Op"=w253, "Assign Val"=w252, "Var Idx"=w261, "Assign Var Idx"=w255, "Priority"=w257, "Delay"=w256) -> (w263:T3)
            n209 = local write "Event Info"(w263) -> ()
          }
          frame #8 {
            n210 = invoke on="XY Graph" class="XYGraph (strict)" method="Reinit To Default"() -> (error out=w559:errorcluster)  [unwired: 3 in, 2 out]
            n211 = local write "Cap Cnt"(0 ("Cap Cnt")) -> ()
            n212 = while {
              tunnel: w561 -> [w565]
              tunnel: w559 -> [_]
              stop <- w570 stop-if-true
              n213 = property on="XY Graph" class="XYGraph (strict)"("Smooth Update"=TRUE) -> ()  [unwired: 2 in, 2 out]
              n214 = event shown="[1] \"Run\": Value Change" {
                selector: _ -> [_ _ _ _ _ _]
                dyn-events: _ -> [_ _ _ _ _ _]
                timeout: 1 -> [_ _ _ _ _ _]
                tunnel: w565 -> [_ _ _ _ w671 _]
                tunnel: [w578 w583 w625 w642 w670 w683] -> w564
                tunnel: [w577 w582 w624 w641 w669 w682] -> w563
                event Timeout {
                  w574 = FALSE ("Visible")
                  n215 = event-data() -> ()  [unwired: 1 in, 3 out]
                  n216 = property on="XY Graph" class="XYGraph (strict)"("LegAutosize"=FALSE ("Legend:Scrollbar Visible")) -> ()  [unwired: 2 in, 2 out]
                  n217 = local read "Status update"() -> (w573:string)
                  n218 = property on="Horizontal Progress Bar" class="Slide (strict)"("Visible"=w574) -> ()  [unwired: 2 in, 2 out]
                  n219 = property on="decimal integer string" class="Str"("Visible"=w574) -> ()  [unwired: 2 in, 2 out]
                  n220 = local write "Status"(w573) -> ()
                  n221 = local read "XY Graph"() -> (w578:cluster{"T":dbl[], dbl[]}[])
                  n222 = local read "Sim Data"() -> (w577:cluster{"times":dbl[], "outputs":dbl[][]})
                  "Horizontal Progress Bar" <- u8 0 ("Horizontal Progress Bar")
                  "decimal integer string" <- ""
                }
                event "Run": Value Change {
                  n223 = event-data() -> ()  [unwired: 1 in, 6 out]
                  n224 = local read "Run"() -> (w581:bool)
                  n225 = case shown="True" w581 {
                    tunnel: [w587 w592] -> w583
                    tunnel: [w586 w591] -> w582
                    tunnel: [FALSE ("Trig Status") FALSE ("Trig Status")] -> w580
                    tunnel: [w584 w595] -> w579
                    frame False {
                      n226 = local read "XY Graph"() -> (w587:cluster{"T":dbl[], dbl[]}[])
                      n227 = local read "Sim Data"() -> (w586:cluster{"times":dbl[], "outputs":dbl[][]})
                      n228 = local read "Status update"() -> (w584:string)
                    }
                    frame True {
                      w597 = "Running simulation" ("Status update")
                      n229 = local read "Parameter info"() -> (w601:string[][])
                      n230 = local read "External Modifiers"() -> (w603:T4[])
                      n231 = local read "Local Parameter Info"() -> (w602:string[][])
                      n232 = local read "SP_for_ODE_Init_Amnt"() -> (w620:string[])
                      n233 = local read "Out_Tot_Param"() -> (w606:string[])
                      n234 = local read "CompID"() -> (w605:string[])
                      n235 = for {
                        tunnel: w603 -> [w622] mode=indexing
                        tunnel: [w621] -> w614 mode=indexing
                        n236 = Unbundle By Name(w622) -> ("Dial"=w621:dbl)
                      }
                      n237 = Fract/Exp String To Number(string=w620) -> (number=w610:dbl[])  [unwired: 3 in, 1 out]
                      n238 = Index Array(array=w601, index (col)=2 ("disabled index (col)")) -> (element=w617:string[])  [unwired: 1 in]
                      n239 = Index Array(array=w602, index (col)=1 ("disabled index (col)")) -> (element=w616:string[])  [unwired: 1 in]
                      n240 = Build Array (concatenate)(w606, w605) -> (w604:string[])
                      n241 = local read "CompSize"() -> (w608:string[])
                      n242 = local write "Status update"(w597) -> ()
                      n243 = local read "Del events after \nexecution"() -> (w589:bool)
                      n244 = local read "Rest_Sp_Init_Amnt"() -> (w590:string[])
                      n245 = local read "Out_X_for_ODE"() -> (w611:string[])
                      n246 = Insert Into Array(array=w617, new element=w616) -> (w609:string[])  [unwired: 1 in]
                      n247 = local read "Ex_Mod_IDs"() -> (w613:string[])
                      n248 = local read "Out_ODE"() -> (w612:string[])
                      n249 = local write "All Param Values"(w609) -> ()
                      n250 = local read "Simulation Parameters"() -> (w600:T1)
                      n251 = Build Array (concatenate)(w609, w608) -> (w607:string[])
                      n252 = local read "All Variables"() -> (w593:string[])
                      n253 = local read "Rest_Sp_IDs"() -> (w588:string[])
                      n254 = local read "Event Info"() -> (w594:T3)
                      n255 = Fract/Exp String To Number(string=w607) -> (number=w615:dbl[])  [unwired: 3 in, 1 out]
                      n256 = call "ODE-VI-28032016.vi"("Param_Value"=w615, "Mod_Value"=w614, "Param_IDs"=w604, "Mod_IDs"=w613, "Initial Conditions for  variables"=w610, "Simulation Parameters"=w600, "ODE Right Hand Side"=w612, "Rest_Sp_IDs"=w588, "Del Events"=w589, "Event Info"=w594, "X (name of variables)"=w611, "All Variables"=w593, "Rest_Sp_Init_Amnt"=w590) -> ("Concentration vs. Time"=w592:cluster{"times":dbl[], dbl[]}[], "Sim Data"=w591:cluster{"times":dbl[], "outputs":dbl[][]})  [unwired: 3 in, 2 out]
                      n257 = Concatenate Strings(w597, " done!" ("string")) -> (w595:string)
                      "Trig Status" <- TRUE ("Trig Status")
                    }
                  }
                  n258 = local write "Status update"(w579) -> ()
                  n259 = local write "Trig Status"(w580) -> ()
                }
                event "Sim Param": Value Change {
                  n260 = event-data() -> ("NewVal"=w626:bool)  [unwired: 1 in, 5 out]
                  n261 = case shown="True" w626 {
                    tunnel: [w629 w633] -> w627
                    tunnel: [w628 w634] -> w623
                    frame False {
                      n262 = local read "Simulation Parameters"() -> (w629:T1)
                      n263 = local read "Status update"() -> (w628:string)
                    }
                    frame True {
                      n264 = flat-sequence {
                        tunnel: [w635] -> w631
                        tunnel: [w638] -> w633
                        tunnel: [w637] -> w632
                        tunnel: w631 -> [w636]
                        tunnel: [w636] -> w630
                        frame #0 {
                          w635 = "Configuring Simulation Settings" ("Status update")
                          n265 = local write "Status"(w635) -> ()
                        }
                        frame #1 {
                          n266 = local read "Simulation Parameters"() -> (w639:T1)
                          n267 = call "ODE Simulation Parameters.vi"("Simulation Parameters In"=w639) -> ("Status"=w637:string, "Simulation Parameters Out"=w638:T1)  [unwired: 3 in]
                        }
                      }
                      n268 = Concatenate Strings(w630, w632) -> (w634:string)
                    }
                  }
                  n269 = local write "Status update"(w623) -> ()
                  n270 = local write "Simulation Parameters"(w627) -> ()
                  n271 = local read "XY Graph"() -> (w625:cluster{"T":dbl[], dbl[]}[])
                  n272 = local read "Sim Data"() -> (w624:cluster{"times":dbl[], "outputs":dbl[][]})
                }
                event "Save Data": Value Change {
                  n273 = event-data() -> ("NewVal"=w643:bool)  [unwired: 1 in, 5 out]
                  n274 = case shown="True" w643 {
                    tunnel: [w644 w645] -> w640
                    frame False {
                      n275 = local read "Status update"() -> (w644:string)
                    }
                    frame True {
                      n276 = stacked-sequence {
                        tunnel: [_ w648] -> w645
                        frame #0 {
                          n277 = local read "Cap Cnt"() -> (w646:i32)
                          n278 = Increment(x=w646) -> (x+1=w647:i32)
                          n279 = local write "Cap Cnt"(w647) -> ()
                        }
                        frame #1 {
                          n280 = local read "Sim Data"() -> (w666:cluster{"times":dbl[], "outputs":dbl[][]})
                          n281 = local read "Cap Cnt"() -> (w660:i32)
                          n282 = Unbundle By Name(w666) -> ("times"=w663:dbl[], "outputs"=w665:dbl[][])
                          n283 = Number To Decimal String(number=w660) -> (decimal integer string=w659:string)  [unwired: 1 in]
                          n284 = Concatenate Strings("Captured Data Set # " ("string"), w659) -> (w656:string)
                          n285 = Insert Into Array(array=w665, index (col)=0 ("disabled index (col)"), new element=w663) -> (w662:dbl[][])  [unwired: 1 in]
                          n286 = Build Array(w656) -> (w655:string[])
                          n287 = Number To Fractional String(number=w662, precision (6)=i16 10) -> (F-format string=w657:string[][])  [unwired: 2 in]
                          n288 = Insert Into Array(array=w657, index (row)=0 ("disabled index (col)"), new element=w655) -> (w654:string[][])  [unwired: 1 in]
                          n289 = local read "DataLog"() -> (w652:path)
                          n290 = call-poly <vilib>:"Write To Spreadsheet File.vi"("append to file? (new file:F)"=TRUE, "2D data"=w654, "file path (dialog if empty)"=w652) -> ()  [unwired: 5 in, 1 out]
                          n291 = Path To String(path=w652) -> (string=w650:string)
                          n292 = Concatenate Strings("Simulation data saved at \"" ("Status update"), w650, "\"" ("string")) -> (w648:string)
                        }
                      }
                    }
                  }
                  n293 = local write "Status update"(w640) -> ()
                  n294 = local read "XY Graph"() -> (w642:cluster{"T":dbl[], dbl[]}[])
                  n295 = local read "Sim Data"() -> (w641:cluster{"times":dbl[], "outputs":dbl[][]})
                }
                event "Capture Graph": Value Change {
                  n296 = event-data() -> ()  [unwired: 1 in, 6 out]
                  n297 = flat-sequence {
                    tunnel: w671 -> [w676]
                    tunnel: [w672] -> w668
                    frame #0 {
                      n298 = invoke on="XY Graph" class="XYGraph (strict)" method="Export Image"("FileType"=enum32{"BMP", "EPS", "EMF", "PICT"}."BMP" ("File Type"), "Target"=enum32{"File", "Clipboard"}."File", "Path"=w676, "Overwrite"=TRUE ("Always Overwrite")) -> ()  [unwired: 4 in, 8 out]
                      n299 = Path To String(path=w676) -> (string=w674:string)
                      n300 = Concatenate Strings("Graph captured and stored at \"" ("string"), w674, ".bmp\"" ("string")) -> (w672:string)
                    }
                  }
                  n301 = local write "Status update"(w668) -> ()
                  n302 = local read "XY Graph"() -> (w670:cluster{"T":dbl[], dbl[]}[])
                  n303 = local read "Sim Data"() -> (w669:cluster{"times":dbl[], "outputs":dbl[][]})
                }
                event "External Modifiers", "Parameter info", "Local Parameter Info": Value Change {
                  n304 = event-data() -> ()  [unwired: 1 in, 6 out]
                  n305 = flat-sequence {
                    tunnel: [w688] -> w683
                    tunnel: [w687] -> w682
                    tunnel: [FALSE ("Trig Status")] -> w681
                    tunnel: [w692] -> w680
                    frame #0 {
                      w694 = "Running simulation" ("Status update")
                      n306 = local read "Parameter info"() -> (w698:string[][])
                      n307 = local read "Local Parameter Info"() -> (w699:string[][])
                      n308 = local read "External Modifiers"() -> (w691:T4[])
                      n309 = local read "SP_for_ODE_Init_Amnt"() -> (w716:string[])
                      n310 = local read "Out_Tot_Param"() -> (w702:string[])
                      n311 = local read "CompID"() -> (w701:string[])
                      n312 = for {
                        tunnel: w691 -> [w718] mode=indexing
                        tunnel: [w717] -> w710 mode=indexing
                        n313 = Unbundle By Name(w718) -> ("Dial"=w717:dbl)
                      }
                      n314 = Fract/Exp String To Number(string=w716) -> (number=w706:dbl[])  [unwired: 3 in, 1 out]
                      n315 = Index Array(array=w698, index (col)=2 ("disabled index (col)")) -> (element=w713:string[])  [unwired: 1 in]
                      n316 = Index Array(array=w699, index (col)=1 ("disabled index (col)")) -> (element=w712:string[])  [unwired: 1 in]
                      n317 = Build Array (concatenate)(w702, w701) -> (w700:string[])
                      n318 = local read "CompSize"() -> (w704:string[])
                      n319 = local write "Status update"(w694) -> ()
                      n320 = local read "Rest_Sp_Init_Amnt"() -> (w686:string[])
                      n321 = local read "Del events after \nexecution"() -> (w685:bool)
                      n322 = local read "Out_X_for_ODE"() -> (w707:string[])
                      n323 = Insert Into Array(array=w713, new element=w712) -> (w705:string[])  [unwired: 1 in]
                      n324 = local read "Ex_Mod_IDs"() -> (w709:string[])
                      n325 = local read "Out_ODE"() -> (w708:string[])
                      n326 = local write "All Param Values"(w705) -> ()
                      n327 = local read "Simulation Parameters"() -> (w697:T1)
                      n328 = local read "Rest_Sp_IDs"() -> (w684:string[])
                      n329 = Build Array (concatenate)(w705, w704) -> (w703:string[])
                      n330 = local read "All Variables"() -> (w689:string[])
                      n331 = local read "Event Info"() -> (w690:T3)
                      n332 = local write "Trig Status"(TRUE ("Trig Status")) -> ()
                      n333 = Fract/Exp String To Number(string=w703) -> (number=w711:dbl[])  [unwired: 3 in, 1 out]
                      n334 = call "ODE-VI-28032016.vi"("Param_Value"=w711, "Mod_Value"=w710, "Param_IDs"=w700, "Mod_IDs"=w709, "Initial Conditions for  variables"=w706, "Simulation Parameters"=w697, "ODE Right Hand Side"=w708, "Rest_Sp_IDs"=w684, "Del Events"=w685, "Event Info"=w690, "X (name of variables)"=w707, "All Variables"=w689, "Rest_Sp_Init_Amnt"=w686) -> ("Concentration vs. Time"=w688:cluster{"times":dbl[], dbl[]}[], "Sim Data"=w687:cluster{"times":dbl[], "outputs":dbl[][]})  [unwired: 3 in, 2 out]
                      n335 = Concatenate Strings(w694, " done!" ("string")) -> (w692:string)
                    }
                  }
                  n336 = local write "Status update"(w680) -> ()
                  n337 = local write "Trig Status"(w681) -> ()
                }
              }
              "XY Graph" <- w564
              "Sim Data" <- w563
              n338 = Wait (ms)(milliseconds to wait=u32 1 ("Simulation Speed (ms)")) -> ()  [unwired: 1 out]
              n339 = global read "Stop ODE.vi" "Stop ODE"() -> (w567:bool)
              n340 = Or(x="Reset", y=w567) -> (x .or. y?=w566:bool)
              n341 = case shown="True" w566 {
                selector: w566 -> [w719 w739]
                tunnel: [w719 w739] -> w570
                tunnel: w565 -> [_ w720]
                frame False {
                }
                frame True {
                  w724 = "Simulation is reset!" ("Status update")
                  n342 = local read "Sim Data"() -> (w730:cluster{"times":dbl[], "outputs":dbl[][]})
                  n343 = global write "Sim status.vi" "Status"(0 ("Status")) -> ()
                  n344 = invoke on="XY Graph" class="XYGraph (strict)" method="Export Image"("FileType"=enum32{"BMP", "EPS", "EMF", "PICT"}."BMP" ("File Type"), "Target"=enum32{"File", "Clipboard"}."File", "Path"=w720, "Overwrite"=TRUE ("Always Overwrite")) -> ()  [unwired: 4 in, 8 out]
                  n345 = Unbundle By Name(w730) -> ("times"=w733:dbl[], "outputs"=w731:dbl[][])
                  n346 = Insert Into Array(array=w731, index (col)=0 ("disabled index (col)"), new element=w733) -> (w734:dbl[][])  [unwired: 1 in]
                  n347 = local write "Status update"(w724) -> ()
                  n348 = local write "Status"(w724) -> ()
                  n349 = Number To Fractional String(number=w734, precision (6)=i16 10) -> (F-format string=w736:string[][])  [unwired: 2 in]
                  n350 = Build Array("Simulation data before simulation reset." ("string")) -> (w737:string[])
                  n351 = local read "DataLog"() -> (w728:path)
                  n352 = Insert Into Array(array=w736, index (row)=0 ("disabled index (col)"), new element=w737) -> (w738:string[][])  [unwired: 1 in]
                  n353 = call-poly <vilib>:"Write To Spreadsheet File.vi"("append to file? (new file:F)"=TRUE, "2D data"=w738, "file path (dialog if empty)"=w728) -> ()  [unwired: 5 in, 1 out]
                }
              }
              n354 = global write "Stop ODE.vi" "Stop ODE"("Reset") -> ()
            }
          }
        }
      }
      frame True {
      }
    }
    "loop" <- w84
  }
  n355 = Not(x=w5) -> (.not. x?=w4:bool)
  n356 = local write "Reset"(w4) -> ()
  n357 = local write "Stop Main"(w4) -> ()
  n358 = disable-structure shown="Enabled" {
    frame Enabled {
      n359 = property on="XY Graph" class="XYGraph (strict)"("LegAutosize"=FALSE ("Legend:Scrollbar Visible")) -> ()  [unwired: 2 in, 2 out]
      n360 = Current VI's Menubar() -> (w752:refnum<k9>)
      n361 = Delete Menu Items(9:w752) -> (3:w751:refnum<k9>)  [unwired: 3 in, 1 out]
      n362 = Insert Menu Items(7:string[] ["File", "Options", "Help"], 9:w751) -> (3:w749:refnum<k9>)  [unwired: 4 in, 2 out]
      n363 = Insert Menu Items(5:"File" ("menu tag"), 7:string[] ["Exit"], 9:w749) -> (3:w743:refnum<k9>)  [unwired: 3 in, 2 out]
      n364 = Insert Menu Items(5:"File" ("menu tag"), 7:string[] ["External Inputs"] ("item tags"), 9:w743) -> (3:w742:refnum<k9>)  [unwired: 3 in, 2 out]
      n365 = Insert Menu Items(5:"Help" ("menu tag"), 7:string[] ["About this Virtual Instrument"] ("item tags"), 9:w742) -> ()  [unwired: 3 in, 3 out]
    }
    frame Disabled {
    }
  }
  n366 = while {
    tunnel: [w756] -> w6
    tunnel: w3 -> [_]
    stop <- w756 stop-if-true
    n367 = Wait Until Next ms Multiple(millisecond multiple=u32 50) -> ()  [unwired: 1 out]
    n368 = property on="XY Graph" class="XYGraph (strict)"("LegAutosize"=FALSE ("Legend:Scrollbar Visible")) -> ()  [unwired: 2 in, 2 out]
    n369 = global write "Stop ODE.vi" "Stop ODE"(FALSE ("Stop ODE")) -> ()
    n370 = event shown="[0] Menu Selection (User)" {
      selector: _ -> [_ _ _ _]
      dyn-events: _ -> [_ _ _ _]
      timeout: 1 -> [_ _ _ _]
      tunnel: [w758 _ TRUE TRUE] -> w756
      tunnel: [w759 _ _ _] -> _
      event Menu Selection (User) {
        n371 = event-data() -> ("ItemTag"=w759:string)  [unwired: 1 in, 6 out]
        n372 = case shown="\"External Inputs\"" w759 {
          tunnel: [_ TRUE _ _] -> w758
          frame "False", Default {
          }
          frame "Exit" {
            w760 = TRUE ("stop")
            n373 = local write "Reset"(w760) -> ()
            n374 = local write "Stop Main"(w760) -> ()
            n375 = global write "Stop ODE.vi" "Stop ODE"(w760) -> ()
          }
          frame "About this Virtual Instrument" {
            n376 = local read "Model Name"() -> (w762:string)
            n377 = call "About ODE VI.vi"("Model Name"=w762) -> ()  [unwired: 11 in]
          }
          frame "External Inputs" {
            n378 = stacked-sequence {
              frame #0 {
                n379 = local write "External Modifiers"(T4[] [] ("Modifiers Array")) -> ()
              }
              frame #1 {
                n380 = local read "Idx of Mod in Sp IDs"() -> (w776:i32[])
                n381 = local read "Rest_Sp_IDs"() -> (w765:string[])
                n382 = local read "Ex_Mod_IDs"() -> (w771:string[])
                n383 = local read "Sp IDs"() -> (w768:string[])
                n384 = local read "Sp_Init_Amnt"() -> (w766:string[])
                n385 = local read "Species Info"() -> (w774:string[][])
                n386 = call "Add-Ex-Mod-Manualy.vi"("In_Sp_Init_Amnt"=w766, "In-Ex_Mod_IDs"=w771, "In-Idx of Mod in Sp IDs"=w776, "Rest_Sp_IDs"=w765, "Sp IDs"=w768) -> ("Out-Rest_Sp_Init_Amnt"=w767:string[], "Out-Ex_Mod_IDs"=w770:string[], "O/p Idx of Mod in Sp IDs"=w769:i32[], "Out_Rest_Sp_IDs"=w764:string[])  [unwired: 3 in]
                n387 = local write "Rest_Sp_Init_Amnt"(w767) -> ()
                n388 = Index Array(array=w774, index (col)=3 ("disabled index (col)")) -> (element=w772:string[])  [unwired: 1 in]
                n389 = local write "Rest_Sp_IDs"(w764) -> ()
                n390 = local write "Ex_Mod_IDs"(w770) -> ()
                n391 = local write "Idx of Mod in Sp IDs"(w769) -> ()
                n392 = for {
                  tunnel: w769 -> [w780] mode=indexing
                  tunnel: w768 -> [w786]
                  tunnel: [w782] -> w775 mode=indexing
                  tunnel: w772 -> [w779]
                  i -> [w784]
                  n393 = local read "External Modifiers"() -> (w785:T4[])
                  n394 = Index Array(array=w786, index=w780) -> (element=w781:string)
                  n395 = Index Array(array=w779, index=w780) -> (element=w778:string)
                  n396 = Fract/Exp String To Number(string=w778) -> (number=w777:dbl)  [unwired: 3 in, 1 out]
                  n397 = Index Array(array=w785, index=w784) -> (element=w783:T4)
                  n398 = Bundle By Name(cluster=w783, "Dial"=w777, "String 2"=w781) -> (w782:T4)
                }
                n399 = local write "External Modifiers"(w775) -> ()
              }
            }
          }
        }
      }
      event Timeout {
        n400 = event-data() -> ()  [unwired: 1 in, 3 out]
        n401 = local read "Trig Status"() -> (w787:bool)
        n402 = case shown="True" w787 {
          frame False {
          }
          frame True {
            w791 = TRUE ("Visible")
            n403 = global read "Sim status.vi" "Status"() -> (w793:i32)
            n404 = Number To Decimal String(number=w793) -> (decimal integer string=w795:string)  [unwired: 1 in]
            n405 = local write "Horizontal Progress Bar"(w793) -> ()
            n406 = Concatenate Strings(w795, " %" ("string")) -> (w792:string)
            n407 = local read "Status update"() -> (w790:string)
            n408 = local write "decimal integer string"(w792) -> ()
            n409 = property on="Horizontal Progress Bar" class="Slide (strict)"("Visible"=w791) -> ()  [unwired: 2 in, 2 out]
            n410 = Concatenate Strings(w790, " ..." ("string")) -> (w789:string)
            n411 = local write "Status"(w789) -> ()
            n412 = property on="decimal integer string" class="Str"("Visible"=w791) -> ()  [unwired: 2 in, 2 out]
          }
        }
      }
      event "Shut Down": Value Change {
        n413 = event-data() -> ()  [unwired: 1 in, 6 out]
        n414 = stacked-sequence {
          frame #0 {
            w797 = TRUE ("stop")
            n415 = local write "Reset"(w797) -> ()
            n416 = local write "Stop Main"(w797) -> ()
            n417 = global write "Stop ODE.vi" "Stop ODE"(w797) -> ()
          }
        }
      }
      event Panel Close {
        w798 = TRUE ("stop")
        n418 = event-data() -> ()  [unwired: 1 in, 4 out]
        n419 = local write "Reset"(w798) -> ()
        n420 = local write "Stop Main"(w798) -> ()
        n421 = global write "Stop ODE.vi" "Stop ODE"(w798) -> ()
      }
    }
  }
  n422 = property class="App"() -> (error out=w9:errorcluster, "App.Kind"=w7:T12)  [unwired: 2 in, 1 out]
  n423 = call <vilib>:"Simple Error Handler.vi"("type of dialog (OK msg:1)"=w8, "error in (no error)"=w9) -> ()  [unwired: 3 in, 5 out]
  n424 = case shown="\"Run Time System\"" w7 {
    tunnel: w6 -> [_ _ _]
    frame "invalid app kind", Default {
    }
    frame "Development System" {
    }
    frame "Run Time System" {
      n425 = control-ref of="This VI"() -> (w802:refnum<vi>)
      n426 = invoke class="VI" method="FP.Close"(reference=w802) -> (reference out=w800:refnum<vi>, error out=w801:errorcluster)  [unwired: 2 in, 1 out]
      n427 = Close Reference(reference=w800, error in (no error)=w801) -> ()  [unwired: 1 out]
    }
  }
